vi "dfd_Group Delay_Adjust Tau.vi"(10 "Coefficients (in)":cluster{"r":dbl[], "theta":dbl[], "offset":dbl}, 11 "Design Info":T1={"p"=2, "freq grid"=[], "d"=[], "weight"=[], "Order"=0, "radius"=1.0}) -> (1 "Error":dbl, 2 "Coefficients (out)":cluster{"r":dbl[], "theta":dbl[], "offset":dbl}, 3 "Design Info (dup)":T1={"p"=2, "freq grid"=[], "d"=[], "weight"=[], "Order"=0, "radius"=1.0})   [LabVIEW 2017, in "NI_DigFilter_Design.lvlib"]
uses:
  <vilib>/addons/Digital Filter Design/NI_DigFilter_Design.lvlib
  <vilib>/addons/Digital Filter Design/_GroupDelay.llb/dfd_Group Delay_Design Info.ctl
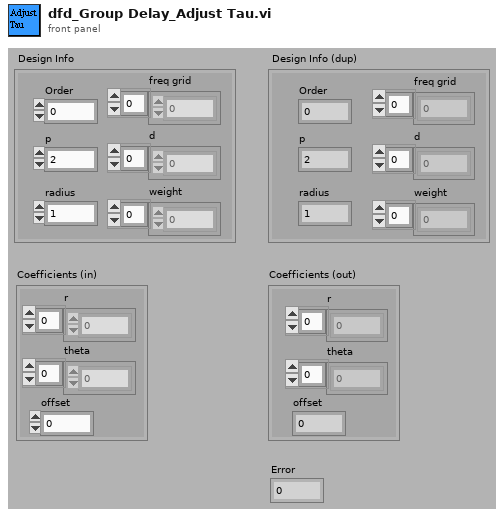
[diagram p1: front panel]
types:
  T1 = typedef "dfd_Group Delay_Design Info.ctl" = cluster{"p":i32, "freq grid":dbl[], "d":dbl[], "weight":dbl[], "Order":i32, "radius":dbl}
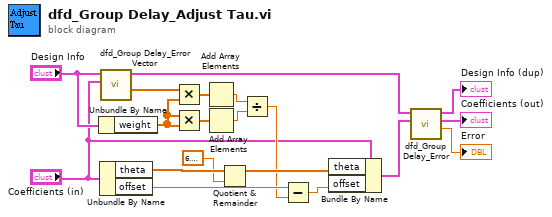
[diagram p0: block diagram]
diagram:
  n1 = Unbundle By Name("Design Info") -> ("weight"=w15:dbl[])
  n2 = Unbundle By Name("Coefficients (in)") -> ("theta"=w19:dbl[], "offset"=w11:dbl)
  n3 = call <vilib>:"dfd_Group Delay_Error Vector.vi"("Coefficients"="Coefficients (in)", "Design Info"="Design Info") -> ("Error"=w14:dbl[], "Design Info (dup)"=w6:T1)  [unwired: 8 out]
  n4 = Multiply(x=w14, y=w15) -> (x*y=w13:dbl[])
  n5 = Multiply(x=w15, y=w15) -> (x*y=w12:dbl[])
  n6 = Add Array Elements(numeric array=w13) -> (sum=w10:dbl)
  n7 = Add Array Elements(numeric array=w12) -> (sum=w9:dbl)
  n8 = Quotient & Remainder(x=w19, y=6.283185307179586) -> (x-y*floor(x/y)=w17:dbl[])  [unwired: 1 out]
  n9 = Divide(x=w10, y=w9) -> (x/y=w8:dbl)
  n10 = Subtract(x=w11, y=w8) -> (x-y=w16:dbl)
  n11 = Bundle By Name(cluster="Coefficients (in)", "theta"=w17, "offset"=w16) -> (w5:cluster{"r":dbl[], "theta":dbl[], "offset":dbl})
  n12 = call <vilib>:"dfd_Group Delay_Error.vi"("Coefficients"=w5, "Design Info"=w6) -> ("Error"=→"Error":dbl, "Coefficients (dup)"=→"Coefficients (out)":cluster{"r":dbl[], "theta":dbl[], "offset":dbl}, "Design Info (dup)"=→"Design Info (dup)":T1)  [unwired: 1 in, 6 out]
